vi "check and update stimulator odor durations (sub-vi).vi"(8 "error in (no error)":errorcluster, 11 "stim. config array refnum":refnum<vi>) -> (0 "error out":errorcluster, 3 "stim. config array refnum out":refnum<vi>, 4 "value error":errorcluster)   [LabVIEW 2021]
uses:
  type-defs/stimulation configuration array (type def).ctl
  type-defs/stimulator configuration line cluster (type def).ctl
  type-defs/port-odor with color cluster (type def).ctl
  type-defs/port-odor ring (type def).ctl
  type-defs/odor color (type def).ctl
  <vilib>/ErrorRing/Error Ring.xnode
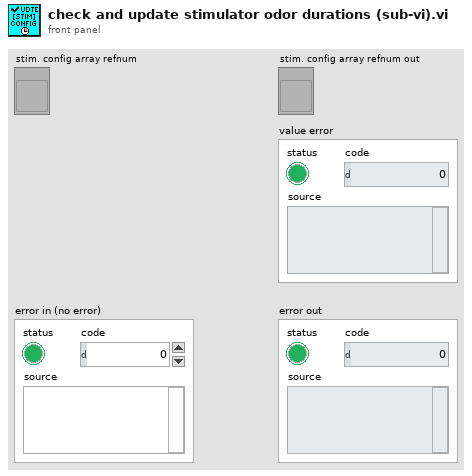
[diagram p1: front panel]
types:
  T1 = typedef "stimulation configuration array (type def).ctl" = T2[]
  T2 = typedef "stimulator configuration line cluster (type def).ctl" = cluster{"description":string, "duration, s":dbl, "left odor":T3, "middle odor":T3, "right odor":T3, "selected?":bool}
  T3 = typedef "port-odor with color cluster (type def).ctl" = cluster{"port-odor ring":T4, "odor color":T5}
  T4 = typedef "port-odor ring (type def).ctl" = u16
  T5 = typedef "odor color (type def).ctl" = u16
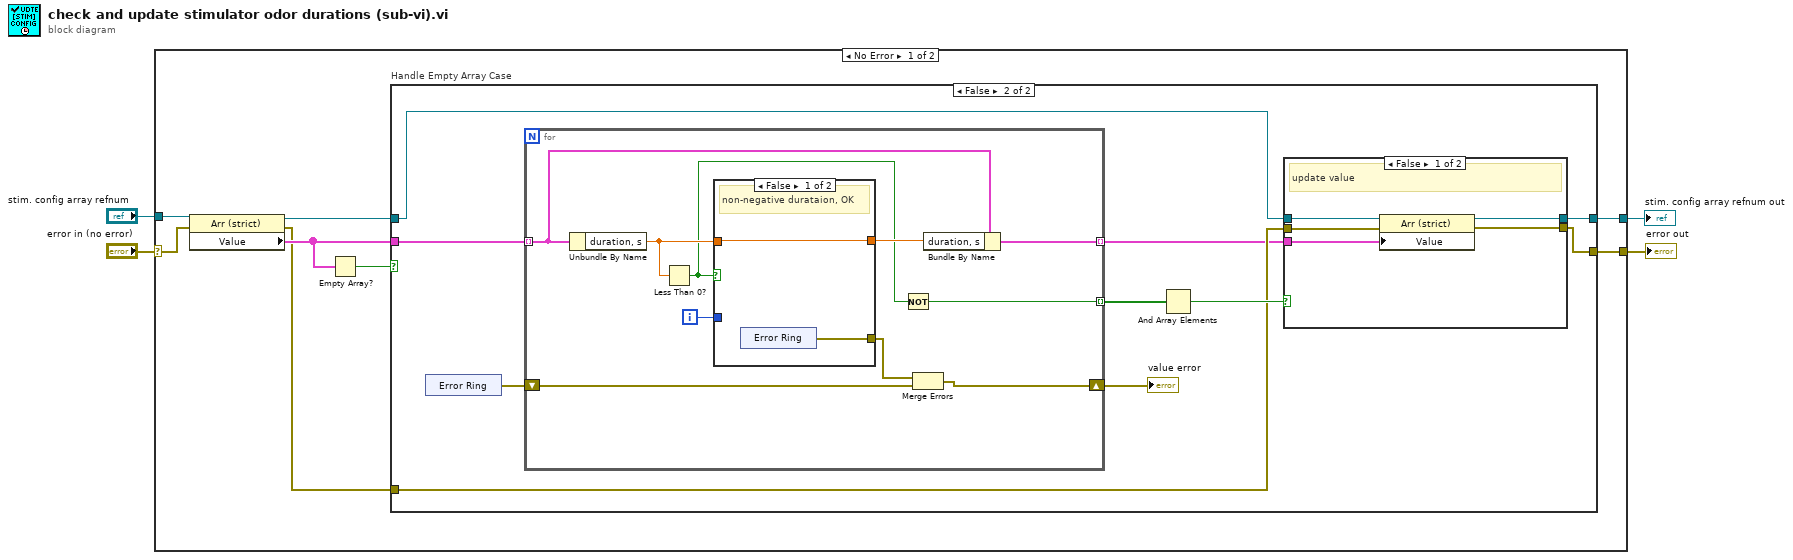
[diagram p0: block diagram]
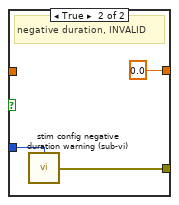
[diagram p4: hidden frame]
diagram:
  n1 = case shown="No Error" "error in (no error)" {
    selector: "error in (no error)" -> [w10 w50]
    tunnel: "stim. config array refnum" -> [w12 w49]
    tunnel: [w9 w49] -> w2
    tunnel: [w8 w50] -> w1
    frame No Error {
      n2 = property class="Arr (strict)"(reference=w12, error in=w10) -> (reference out=w11:refnum<vi>, error out=w6:errorcluster, "Value"=w7:T1)
      n3 = Empty Array?(array=w7) -> (empty?=w5:bool)
      n4 = case "Handle Empty Array Case" shown="False" w5 {
        tunnel: w11 -> [w14 w19]
        tunnel: [w14 w17] -> w9
        tunnel: [w13 w16] -> w8
        tunnel: w7 -> [_ w24]
        tunnel: w6 -> [w13 w18]
        frame True {
        }
        frame False {
          n5 = xnode "Error Ring"() -> ("error out"=w22:errorcluster)
          n6 = for {
            tunnel: w24 -> [w42] mode=indexing
            shift-right: [w34] -> w23
            shift-left: w22 -> [w35]
            tunnel: [w41] -> w15 mode=indexing
            tunnel: [w38] -> w21 mode=indexing
            i -> [w36]
            n7 = Unbundle By Name(w42) -> ("duration, s"=w40:dbl)
            n8 = Less Than 0?(x=w40) -> (x < 0?=w37:bool)
            n9 = case shown="False" w37 {
              tunnel: w40 -> [w44 _]
              tunnel: [w44 0.0 ("duration, s")] -> w39
              tunnel: [w43 w47] -> w33
              tunnel: w36 -> [_ w46]
              frame False {
                # "non-negative durataion, OK"
                n10 = xnode "Error Ring"() -> ("error out"=w43:errorcluster)
              }
              frame True {
                # "negative duration, INVALID"
                n11 = call "stim config negative duration warning (sub-vi).vi"("entry line index (-1, no entry index)"=w46) -> ("error"=w47:errorcluster)  [unwired: 3 in]
              }
            }
            n12 = Not(x=w37) -> (.not. x?=w38:bool)
            n13 = Merge Errors(w33, w35) -> (w34:errorcluster)
            n14 = Bundle By Name(cluster=w42, "duration, s"=w39) -> (w41:T2)
          }
          "value error" <- w23
          n15 = And Array Elements(Boolean array=w21) -> (logical AND=w20:bool)
          n16 = case shown="False" w20 {
            tunnel: w19 -> [w29 w31]
            tunnel: w18 -> [w27 w30]
            tunnel: [w25 w31] -> w17
            tunnel: [w26 w30] -> w16
            tunnel: w15 -> [w28 _]
            frame False {
              # "update value"
              n17 = property class="Arr (strict)"(reference=w29, error in=w27, "Value"=w28) -> (reference out=w25:refnum<vi>, error out=w26:errorcluster)
            }
            frame True {
              # "no change to value"
            }
          }
        }
      }
    }
    frame Error {
    }
  }
  "stim. config array refnum out" <- w2
  "error out" <- w1
